vi "Determine if Client Assigns.vi"(10 "Server Value In":T1, 11 "Name":string) -> (2 "Assignment Value":T1, 3 "Update Server":bool)   [LabVIEW 2017]
uses:
  <vilib>/Rock Robotics/Network Tables/Field Data.ctl
  <vilib>/Rock Robotics/Network Tables/Field Type.ctl
  <vilib>/Rock Robotics/Network Tables/Sequence.ctl
  <vilib>/Rock Robotics/Network Tables/Make Table Operation.ctl
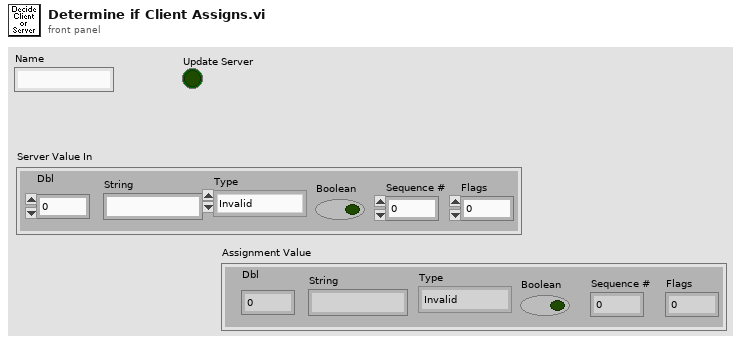
[diagram p1: front panel]
types:
  T1 = typedef "Field Data.ctl" = cluster{"Dbl":dbl, "String":string, "Type":T2, "Boolean":bool, "Sequence #":T3, "Flags":u8}
  T2 = typedef "Field Type.ctl" = enum8{"Invalid", "Bool", "Numeric", "String", "Raw", "Boolean Array", "Numeric Array", "String Array", "RPC"}
  T3 = typedef "Sequence.ctl" = u16
  T4 = enum16{"Update Field", "Read Field", "Assign Field", "Remove All", "Set Persistence", "Clear Persistence"}
  T5 = typedef "Make Table Operation.ctl" = enum16{"Get or Add Field", "Get Field or Add Temp", "Replace Temp ID", "Get Field ID - No Add", "Get Table Field IDs", "Get Field ID Info", "Move Field to Temp", "Validate", "Remove Field", "Remove All"}
  T6 = typedef "Field ID.ctl" = i32
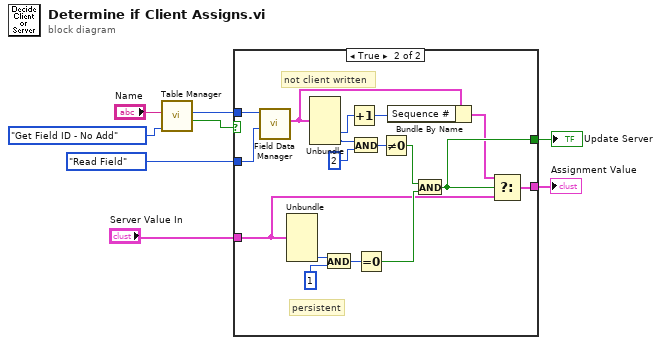
[diagram p0: block diagram]
diagram:
  n1 = call <vilib>:"Table Manager.vi"("Operation"=Make_Table_Operation."Get Field ID - No Add", "Entry Name"="Name") -> ("Success"=w5:bool, "Entry ID"=w8:T6)  [unwired: 6 in, 2 out]
  n2 = case shown="True" w5 {
    tunnel: w8 -> [_ w26]
    tunnel: T4."Read Field" ("Operation") -> [_ w25]
    tunnel: "Server Value In" -> [w9 w15]
    tunnel: [w9 w20] -> w2
    tunnel: [_ w14] -> w1
    frame False {
    }
    frame True {
      # "not client written"
      # "persistent"
      n3 = call <vilib>:"Field Data Manager.vi"("Operation"=w25, "Field ID"=w26) -> ("Field Value Out"=w11:T1)  [unwired: 8 in, 1 out]
      n4 = Unbundle(w15) -> ("Flags"=w21:u8)  [unwired: 5 out]
      n5 = Unbundle(w11) -> ("Sequence #"=w13:T3, "Flags"=w23:u8)  [unwired: 4 out]
      n6 = And(x=w21, y=1) -> (x .and. y?=w18:i32)
      n7 = Increment(x=w13) -> (x+1=w12:T3)
      n8 = And(x=w23, y=2) -> (x .and. y?=w19:i32)
      n9 = Equal To 0?(x=w18) -> (x = 0?=w17:bool)
      n10 = Not Equal To 0?(x=w19) -> (x != 0?=w16:bool)
      n11 = Bundle By Name(cluster=w11, "Sequence #"=w12) -> (w10:T1)
      n12 = And(x=w16, y=w17) -> (x .and. y?=w14:bool)
      n13 = Select(t=w10, s=w14, f=w15) -> (s? t:f=w20:T1)
    }
  }
  "Assignment Value" <- w2
  "Update Server" <- w1
